vi "Range.vi"(8 "error in (no error)":errorcluster, 10 "Range":u32(ring) items=["Auto", "Lowest", "2", "3", "4", "5", "6", "7", "Highest"], 11 "VISA resource name":refnum<visa-resource-name>) -> (0 "error out":errorcluster, 3 "VISA resource name out":refnum<visa-resource-name>)   [LabVIEW 2013, in "Newport 1830-C.lvlib"]
doc: "0=AutoRange\n1=Lowest manual singal range (highest amplifier gain)\n'''\n'''\n'''\n8=highest manual signal range (lowest amplifier gain)"
uses:
  Newport 1830-C.lvlib
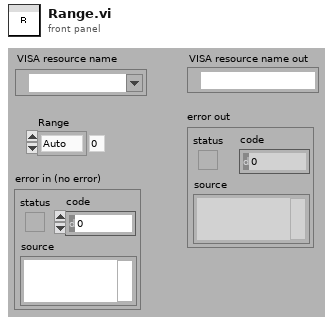
[diagram p1: front panel]
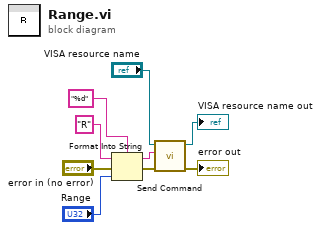
[diagram p0: block diagram]
diagram:
  n1 = Format Into String(format string="%d", initial string="R" ("command"), error in="error in (no error)", "Range") -> (resulting string=w5:string, error out=w6:errorcluster)
  n2 = call "Send Command.vi"("error in (no error)"=w6, "write buffer"=w5, "VISA resource name In"="VISA resource name") -> ("error out"=→"error out":errorcluster, "VISA resource name out"=→"VISA resource name out":refnum<visa-resource-name>)  [unwired: 7 in]
